vi "main.vi"() -> ()   [LabVIEW 2017]
uses:
  <vilib>/sound2/lvsound2.llb/Sound Data Format.ctl
  mainVIs/States.ctl
  <vilib>/sound2/lvsound2.llb/Sound Input Task ID.ctl
  <vilib>/sound2/lvsound2.llb/Sampling Mode.ctl
  <vilib>/sound2/lvsound2.llb/Sound Input Read (DBL).vi
panel:
  out "Enum":T1
  out "Time Signal":waveform(dbl)[](graph)
  in  "number of samples/ch":i32=100000
  in  "sound format":T2={"sample rate (S/s)"=22050.0, "number of channels"=2, "bits per sample"=16}
  in  "?":bool
  in  "stop":bool
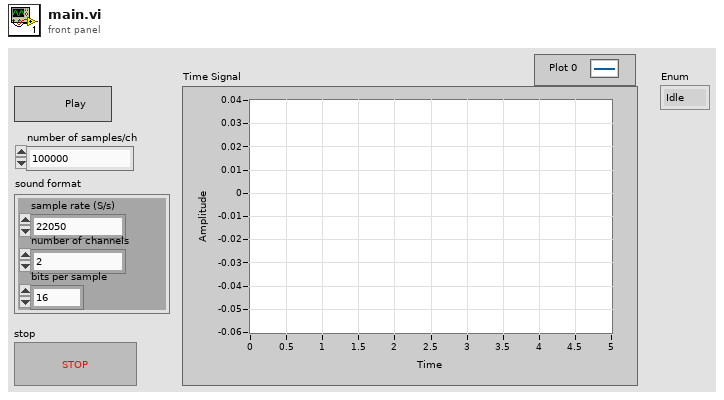
[diagram p1: front panel]
types:
  T1 = typedef "States.ctl" = enum16{"Idle", "Initialization", "Acquisition", "Finish"}
  T2 = typedef "Sound Data Format.ctl" = cluster{"sample rate (S/s)":dbl, "number of channels":i32, "bits per sample":i32}
  T3 = typedef "Sound Input Task ID.ctl" = u32
  T4 = typedef "Sampling Mode.ctl" = i32
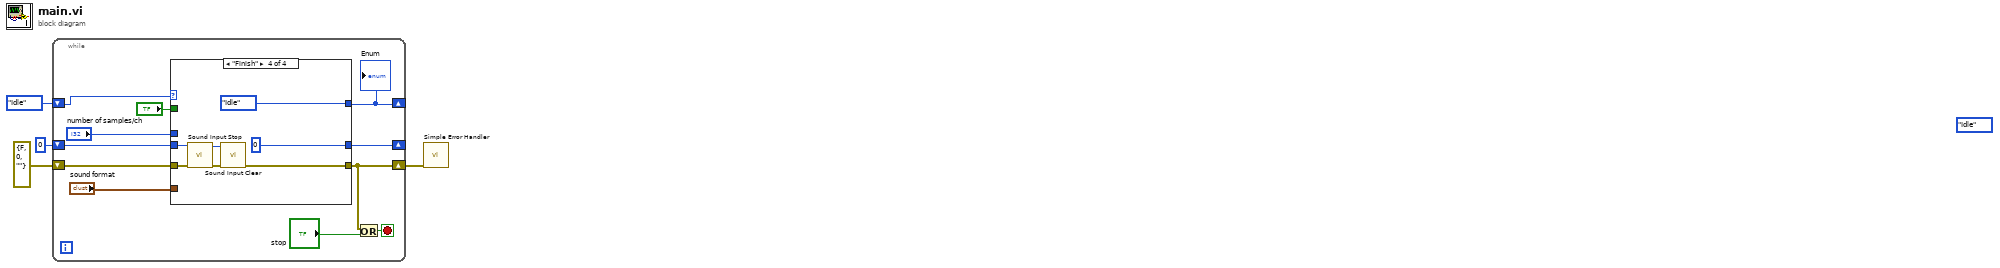
[diagram p0: block diagram]
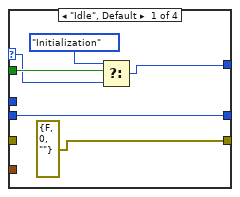
[diagram p2: hidden frame]
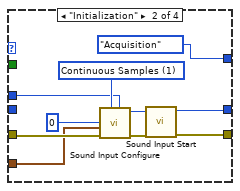
[diagram p3: hidden frame]
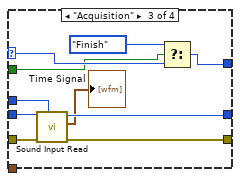
[diagram p4: hidden frame]
diagram:
  (unwired) States."Idle"
  n1 = while {
    shift-right: [w14] -> _
    shift-left: States."Idle" ("Enum") -> [w15]
    shift-right: [w6] -> w3
    shift-left: errorcluster {"status"=FALSE, "code"=0, "source"=""} ("error out") -> [w12]
    shift-right: [w9] -> _
    shift-left: T3 0 ("task ID out") -> [w8]
    stop <- w7 stop-if-true
    n2 = case shown="\"Finish\"" w15 {
      selector: w15 -> [w18 _ w34 _]
      tunnel: [w21 States."Acquisition" ("Enum") w41 States."Idle" ("Enum")] -> w14
      tunnel: "?" -> [w19 _ w32 _]
      tunnel: [errorcluster {"status"=FALSE, "code"=0, "source"=""} ("error out") w24 w37 w43] -> w6
      tunnel: w12 -> [_ w30 w39 w46]
      tunnel: "sound format" -> [_ w29 _ _]
      tunnel: "number of samples/ch" -> [_ w27 w36 _]
      tunnel: [w16 w23 w38 T3 0 ("task ID out")] -> w9
      tunnel: w8 -> [w16 _ w40 w47]
      frame "Idle", Default {
        n3 = Select(t=States."Initialization" ("Enum"), s=w19, f=w18) -> (s? t:f=w21:T1)
      }
      frame "Initialization" {
        w28 = T4 1 items=["Finite Samples", "Continuous Samples"] ("sample mode")
        n4 = call <vilib>:"Sound Input Configure.vi"("number of samples/ch"=w27, "sample mode"=w28, "error in (no error)"=w30, "sound format"=w29, "device ID"=u32 0) -> ("error out"=w25:errorcluster, "task ID"=w26:T3)  [unwired: 5 in]
        n5 = call <vilib>:"Sound Input Start.vi"("error in (no error)"=w25, "task ID"=w26) -> ("error out"=w24:errorcluster, "task ID out"=w23:T3)  [unwired: 8 in]
      }
      frame "Acquisition" {
        n6 = call-poly <vilib>:"Sound Input Read.vi"("number of samples/ch"=w36, "error in (no error)"=w39, "task ID"=w40) -> ("error out"=w37:errorcluster, "data"=→"Time Signal":waveform(dbl)[], "task ID out"=w38:T3)  [unwired: 6 in]
        n7 = Select(t=States."Finish" ("Enum"), s=w32, f=w34) -> (s? t:f=w41:T1)
      }
      frame "Finish" {
        n8 = call <vilib>:"Sound Input Stop.vi"("error in (no error)"=w46, "task ID"=w47) -> ("error out"=w44:errorcluster, "task ID out"=w45:T3)  [unwired: 8 in]
        n9 = call <vilib>:"Sound Input Clear.vi"("error in (no error)"=w44, "task ID"=w45) -> ("error out"=w43:errorcluster)  [unwired: 9 in]
      }
    }
    "Enum" <- w14
    n10 = Or(x=w6, y="stop") -> (x .or. y?=w7:bool)
  }
  n11 = call <vilib>:"Simple Error Handler.vi"("error in (no error)"=w3) -> ()  [unwired: 4 in, 5 out]
